vi "LinxAnalogRead.vi"(8 "Error In":errorcluster, 10 "Channels":u8[](array[numeric]), 11 "LINX Resource":T1) -> (0 "Error Out":errorcluster, 1 "AI Ref":dbl, 2 "AI Values":dbl[](array[numeric]), 3 "LINX Resource":T1)   [LabVIEW 2020, in "LMH-LINX.lvlib" / "Local IO.lvlib"]
uses:
  <vilib>/MakerHub/LINX/Private/Local IO/Local IO.lvlib
  <vilib>/MakerHub/LINX/Private/Type Defs/LINX Ref.ctl
  <vilib>/MakerHub/LINX/Private/Type Defs/Platform.ctl
  <vilib>/MakerHub/LINX/Private/Type Defs/Interface.ctl
  <vilib>/MakerHub/LINX/Private/Device/Type Defs/LINX Device Config.ctl
  <vilib>/MakerHub/LINX/Private/Device/Type Defs/TCP Config.ctl
  <vilib>/MakerHub/LINX/Private/Device/Type Defs/Channels.ctl
  <vilib>/MakerHub/LINX/Resources/liblinxdevice.dll
  <vilib>/MakerHub/LINX/LMH-LINX.lvlib
  <vilib>/MakerHub/LINX/Private/Device/Device.lvlib
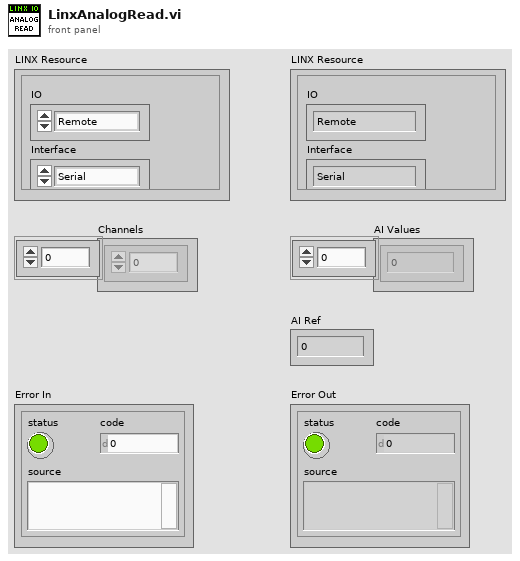
[diagram p1: front panel]
types:
  T1 = typedef "LMH-LINX.lvlib/LINX Ref.ctl" = cluster{"IO":T2, "Interface":T3, "LINX Device Config":T4}
  T2 = typedef "LMH-LINX.lvlib/Platform.ctl" = enum16{"Remote", "Local"}
  T3 = typedef "LMH-LINX.lvlib/Interface.ctl" = enum16{"Serial", "TCP"}
  T4 = typedef "LMH-LINX.lvlib/Device.lvlib/LINX Device Config.ctl" = cluster{"Interface":T3, "COM Port":refnum<visa-resource-name>, "TCP Configuration":T5, "Device Family":u8, "Device ID":u8, "Device Name":string, "TCP Ref":refnum<k5>, "Channels":T6}
  T5 = typedef "LMH-LINX.lvlib/Device.lvlib/TCP Config.ctl" = cluster{"IP Address":string, "Port":u16}
  T6 = typedef "LMH-LINX.lvlib/Channels.ctl" = cluster{"DI":u8[], "DO":u8[], "AI":u8[], "AO":u8[], "PWM":u8[], "QE":u8[], "UART":u8[], "I2C 2":u8[], "SPI":u8[], "CAN":u8[], "Servo":u8[], "AI Ref (V)":dbl, "AI Resolution (Bits)":u8, "AO Ref (V)":dbl, "AO Resolution (Bits)":u8}
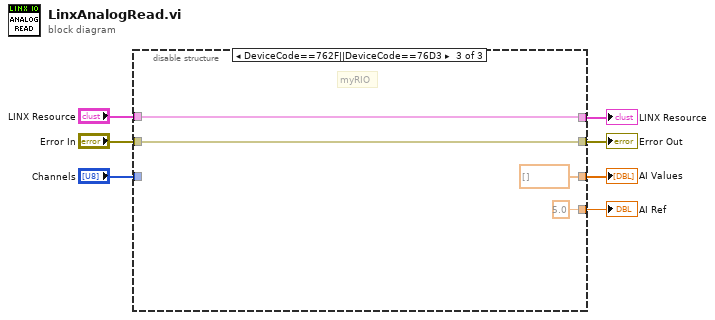
[diagram p0: block diagram]
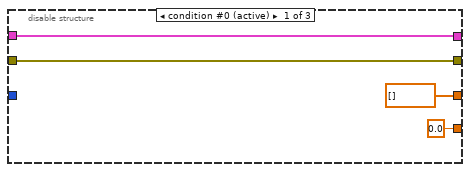
[diagram p2: hidden frame]
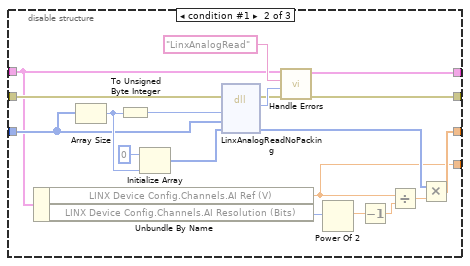
[diagram p3: hidden frame]
diagram:
  n1 = disable-structure shown="DeviceCode==762F||DeviceCode==76D3" {
    disable-tunnel: [w11 w23 w34] -> w7
    disable-tunnel: [w10 w22 w33] -> w6
    disable-tunnel: "LINX Resource" -> [w11 w19 w34]
    disable-tunnel: "Error In" -> [w10 w21 w33]
    disable-tunnel: "Channels" -> [_ w20 _]
    disable-tunnel: [dbl[] [] ("AI Values") w17 dbl[] [] ("AI Values")] -> w2
    disable-tunnel: [0.0 ("AI Ref") w16 5.0 ("AI Ref")] -> w1
    frame condition #0 (active) {
    }
    frame condition #1 {
      n2 = Unbundle By Name(w19) -> ("LINX Device Config.Channels.AI Ref (V)"=w16:dbl, "LINX Device Config.Channels.AI Resolution (Bits)"=w15:u8)
      n3 = Array Size(array=w20) -> (size(s)=w25:i32)
      n4 = To Unsigned Byte Integer(number=w25) -> (unsigned 8bit integer=w24:u8)
      n5 = Initialize Array(u32 0 ("element"), w25) -> (w30:u32[])
      n6 = dll-call lib="C:/Program Files (x86)/National Instruments/LabVIEW 2020/vi.lib/MakerHub/LINX/Resources/liblinxdevice.*" fn="LinxAnalogReadNoPacking"(error in=w21, "numChans"=w24, "channels"=w20, "values"=w30) -> (error out=w26:errorcluster, "LinxStatus"=w27:i32, "values"=w18:u32[])  [unwired: 4 in, 1 out]
      n7 = call <vilib>:"Handle Errors.vi"("Error In"=w26, "LinxStatus"=w27, "Function Name"="LinxAnalogRead", "LINX Resource"=w19) -> ("Error Out"=w22:errorcluster, "LINX Resource"=w23:T1)  [unwired: 6 in]
      n8 = Power Of 2(x=w15) -> (2^x=w12:dbl)
      n9 = Decrement(x=w12) -> (x-1=w14:dbl)
      n10 = Divide(x=w16, y=w14) -> (x/y=w13:dbl)
      n11 = Multiply(x=w18, y=w13) -> (x*y=w17:dbl[])
    }
    frame condition #2 {
      # "myRIO"
    }
  }
  "Error Out" <- w6
  "LINX Resource" <- w7
  "AI Values" <- w2
  "AI Ref" <- w1
